vi "Handle Packet Identifier.vi"(8 "error in (no error)":errorcluster, 10 "Incoming Packets":u8[](array[numeric]) format="%08b", 11 "ControlPacket in":refnum<class "ControlPacket.lvclass">) -> (0 "error out":errorcluster, 1 "Identifier Complete?":bool=TRUE, 2 "Remaining Packets":u8[](array[numeric]) format="%08b", 3 "ControlPacket out":refnum<class "ControlPacket.lvclass">)   [LabVIEW 2013, in "MQTT_Control_Packets.lvlib" / "ControlPacket.lvclass"]
uses:
  ControlPacket.lvclass
  ControlPacket.lvclass/ControlPacket.ctl
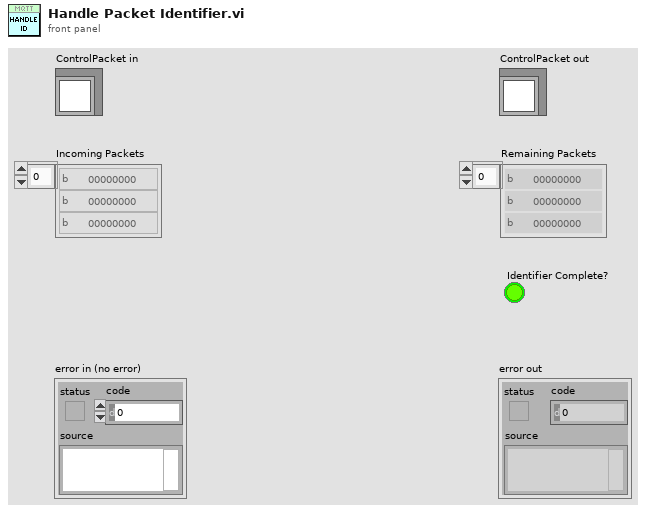
[diagram p1: front panel]
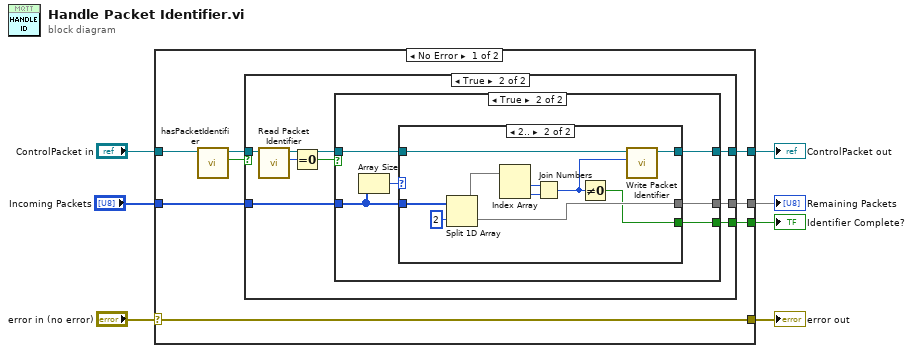
[diagram p0: block diagram]
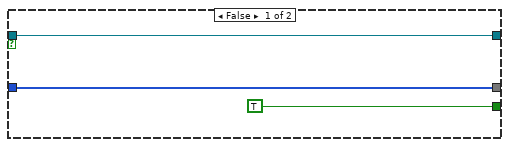
[diagram p2: hidden frame]
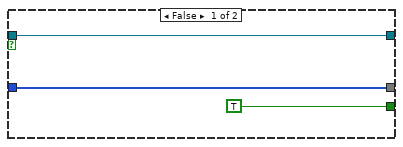
[diagram p3: hidden frame]
diagram:
  n1 = case shown="No Error" "error in (no error)" {
    selector: "error in (no error)" -> [w15 w50]
    tunnel: [w15 w50] -> w6
    tunnel: [w14 w49] -> w4
    tunnel: "ControlPacket in" -> [w10 w49]
    tunnel: "Incoming Packets" -> [w11 w48]
    tunnel: [w13 w48] -> w2
    tunnel: [w12 _] -> w1
    frame No Error {
      n2 = call-dynamic "hasPacketIdentifier.vi"("ControlPacket in"=w10) -> ("Has Packet Identifier"=w8:bool, "ControlPacket out"=w9:refnum<class "ControlPacket.lvclass">)  [unwired: 9 in]
      n3 = case shown="True" w8 {
        tunnel: [w18 w26] -> w14
        tunnel: [w17 w25] -> w13
        tunnel: [TRUE w23] -> w12
        tunnel: w11 -> [w17 w21]
        tunnel: w9 -> [w18 w20]
        frame False {
        }
        frame True {
          n4 = call "Read Packet Identifier.vi"("ControlPacket in"=w20) -> ("Packet Identifier"=w22:u16, "ControlPacket out"=w24:refnum<class "ControlPacket.lvclass">)  [unwired: 9 in]
          n5 = Equal To 0?(x=w22) -> (x = 0?=w19:bool)
          n6 = case shown="True" w19 {
            tunnel: w24 -> [w29 w35]
            tunnel: [w29 w34] -> w26
            tunnel: w21 -> [w28 w32]
            tunnel: [w28 w33] -> w25
            tunnel: [TRUE w30] -> w23
            frame False {
            }
            frame True {
              n7 = Array Size(array=w32) -> (size(s)=w31:i32)
              n8 = case shown="2.." w31 {
                tunnel: w35 -> [w37 w47]
                tunnel: [w37 w46] -> w34
                tunnel: [w36 w45] -> w33
                tunnel: w32 -> [w36 w40]
                tunnel: [_ w39] -> w30
                frame Default {
                }
                frame 2.. {
                  n9 = Split 1D Array(array=w40, index=2 ("length")) -> (first subarray=w38:u8[], second subarray=w45:u8[])
                  n10 = Index Array(array=w38) -> (element #1=w43:u8, element #2=w44:u8)  [unwired: 2 in]
                  n11 = Join Numbers(hi=w43, lo=w44) -> ((hi.lo)=w42:u16)
                  n12 = Not Equal To 0?(x=w42) -> (x != 0?=w39:bool)
                  n13 = call "Write Packet Identifier.vi"("Packet Identifier"=w42, "ControlPacket in"=w47) -> ("ControlPacket out"=w46:refnum<class "ControlPacket.lvclass">)  [unwired: 9 in]
                }
              }
            }
          }
        }
      }
    }
    frame Error {
    }
  }
  "error out" <- w6
  "ControlPacket out" <- w4
  "Remaining Packets" <- w2
  "Identifier Complete?" <- w1
